vi "results.vi"(11 "Quantities":T1[](array[typedef])) -> (3 "Quantities out":T1[](array[typedef]))   [LabVIEW 2013]
uses:
  qwtb_lvlib/TD Quantity.ctl
  <vilib>/Utility/xml.llb/Write to XML File(string).vi
  <vilib>/Utility/xml.llb/Read From XML File(string).vi
panel:
  in  "load Q":bool
  in  "save Q":bool
  in  "Q list curr value":i32
  in  "Q list":i32(listbox) caption="Input Quantities"
  in  "quit":bool
  out "Q name":string caption="Name of Quantity:"
  in  "Q type":enum32{"Scalar", "Vector"}(tab)
  out "scalar dof":dbl=1.0 caption="DoF"
  out "scalar value":dbl=1.0 caption="Value"
  out "scalar unc":dbl=1.0 caption="Uncertainty"
  in  "set dof same as 1st":bool
  out "vector dof":dbl[](array[numeric]) caption="DoF"
  out "vector value":dbl[](array[numeric]) caption="Value"
  out "vector unc":dbl[](array[numeric]) caption="Uncertainty"
  out "Value Graph":dbl[](graph)
  in  "load csv":bool
  # "Results"
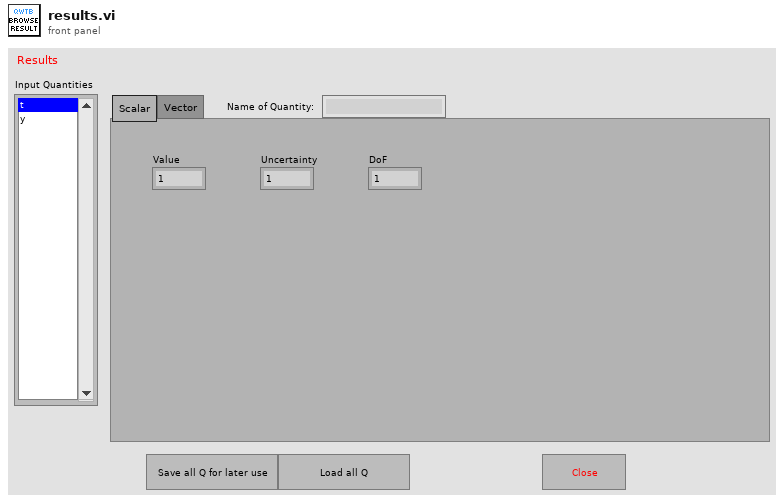
[diagram p1: front panel]
types:
  T1 = typedef "TD Quantity.ctl" = cluster{"Name":string, "Value":dbl[], "Uncertainty":dbl[][], "Degrees of\nFreedom":dbl[]}
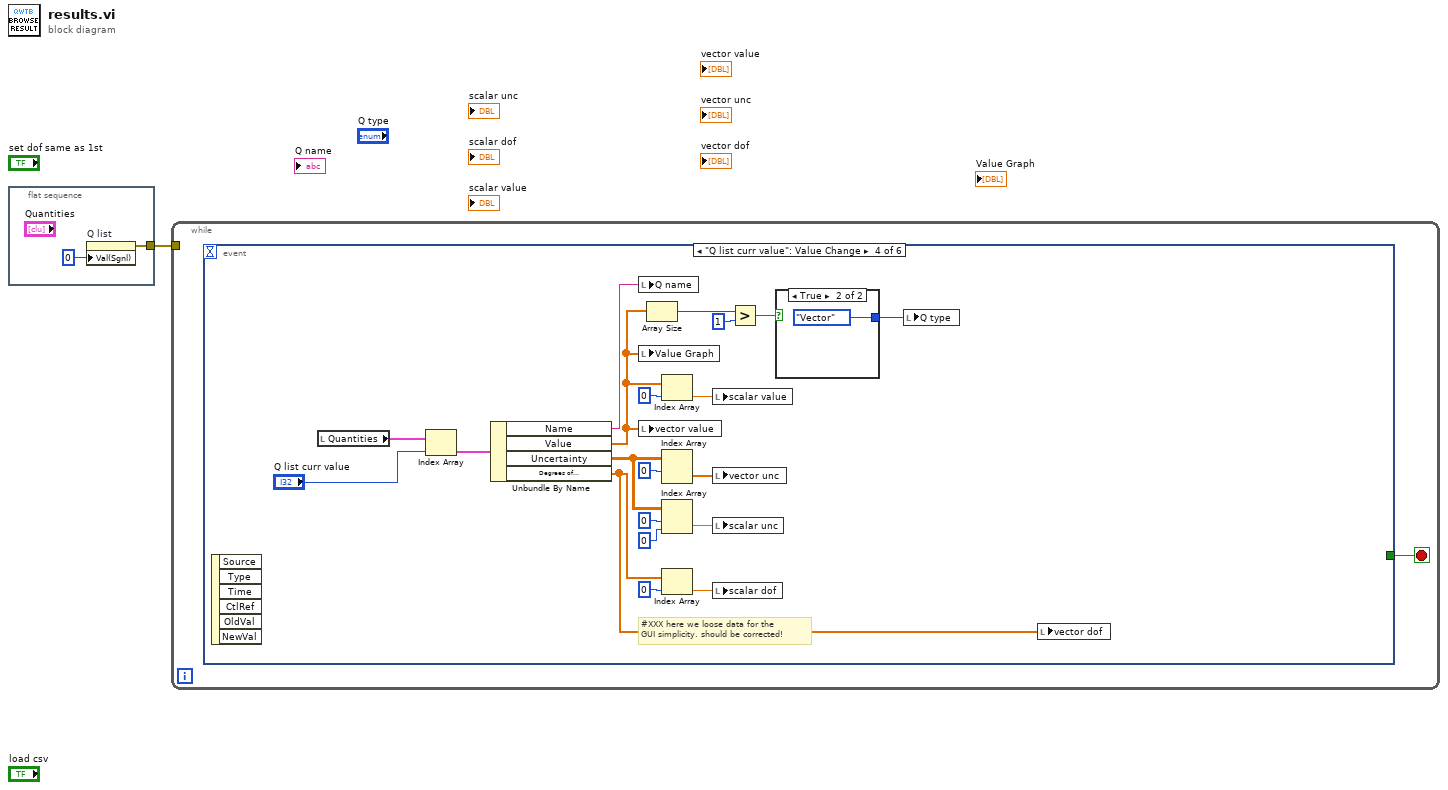
[diagram p0: block diagram]
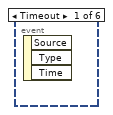
[diagram p2: hidden frame]
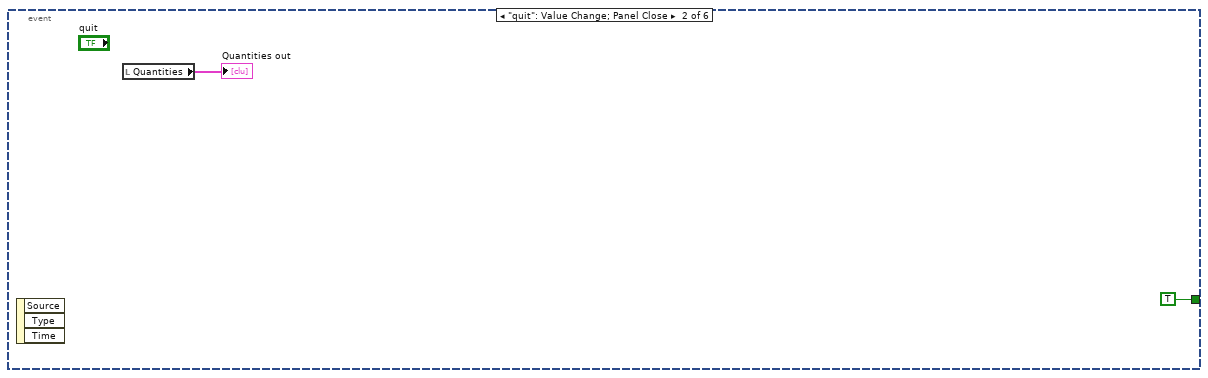
[diagram p3: hidden frame]
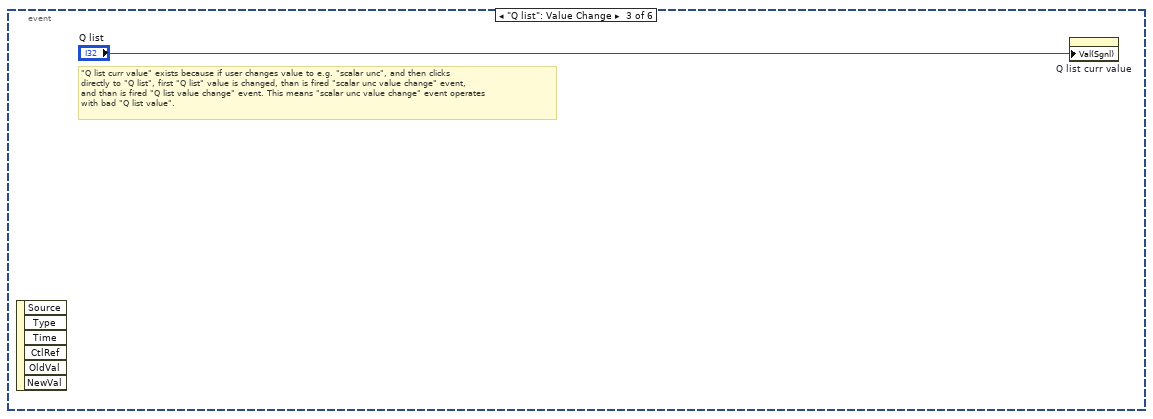
[diagram p4: hidden frame]
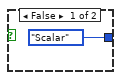
[diagram p5: hidden frame]
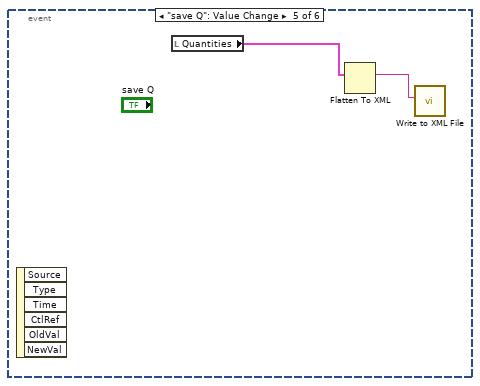
[diagram p6: hidden frame]
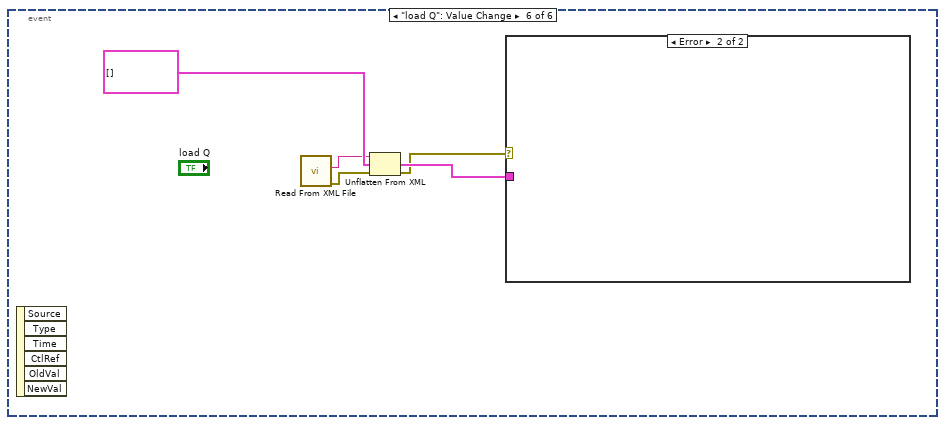
[diagram p7: hidden frame]
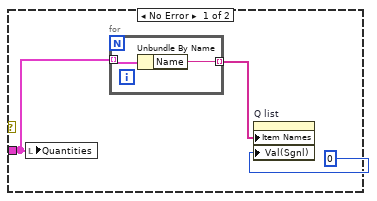
[diagram p8: hidden frame]
diagram:
  n1 = flat-sequence {
    tunnel: [w2] -> w1
    frame #0 {
      n2 = property on="Q list" class="LstBox (strict)"("Val(Sgnl)"=0 ("Value (Signaling)")) -> (error out=w2:errorcluster)  [unwired: 2 in, 1 out]
    }
  }
  n3 = while {
    tunnel: w1 -> [_]
    stop <- w4 stop-if-true
    n4 = event shown="[3] \"Q list curr value\": Value Change" {
      selector: _ -> [_ _ _ _ _ _]
      dyn-events: _ -> [_ _ _ _ _ _]
      timeout: _ -> [_ _ _ _ _ _]
      tunnel: [_ TRUE _ _ _ _] -> w4
      event Timeout {
        n5 = event-data() -> ()  [unwired: 1 in, 3 out]
      }
      event "quit": Value Change; Panel Close {
        n6 = event-data() -> ()  [unwired: 1 in, 3 out]
        n7 = local read "Quantities"() -> (→"Quantities out":T1[])
      }
      event "Q list": Value Change {
        # "\"Q list curr value\" exists because if user changes value to e.g. \"scalar unc\", and then clicks\ndirectly to \"Q list\", first \"Q list\" value is changed, than is fired \"scalar unc value change\" event,\nand than is fired \"Q list value change\" event. This means \"scalar unc value change\" event operates\nwith bad \"Q list value\"."
        n8 = event-data() -> ()  [unwired: 1 in, 6 out]
        n9 = property on="Q list curr value" class="DigNum (strict)"("Val(Sgnl)"="Q list") -> ()  [unwired: 2 in, 2 out]
      }
      event "Q list curr value": Value Change {
        # "#XXX here we loose data for the\nGUI simplicity. should be corrected!"
        n10 = event-data() -> ()  [unwired: 1 in, 6 out]
        n11 = local read "Quantities"() -> (w25:T1[])
        n12 = Index Array(array=w25, index="Q list curr value") -> (element=w27:T1)
        n13 = Unbundle By Name(w27) -> ("Name"=w26:string, "Value"=w11:dbl[], "Uncertainty"=w12:dbl[][], "Degrees of\nFreedom"=w8:dbl[])
        n14 = local write "Q name"(w26) -> ()
        n15 = local write "Value Graph"(w11) -> ()
        n16 = local write "vector value"(w11) -> ()
        n17 = Array Size(array=w11) -> (size(s)=w24:i32)
        n18 = Index Array(array=w11, index=0) -> (element=w13:dbl)
        n19 = Index Array(array=w12, index (row)=0) -> (element=w19:dbl[])  [unwired: 1 in]
        n20 = Index Array(array=w12, index (row)=0, index (col)=0 ("disabled index (col)")) -> (element=w16:dbl)
        n21 = Index Array(array=w8, index=0) -> (element=w9:dbl)
        n22 = local write "scalar value"(w13) -> ()
        n23 = local write "vector unc"(w19) -> ()
        n24 = local write "scalar unc"(w16) -> ()
        n25 = local write "scalar dof"(w9) -> ()
        n26 = Greater?(x=w24, y=1) -> (0:w22:bool)
        n27 = case shown="True" w22 {
          tunnel: [enum32{"Scalar", "Vector"}."Scalar" ("Quantity type") enum32{"Scalar", "Vector"}."Vector" ("Quantity type")] -> w21
          frame False {
          }
          frame True {
          }
        }
        n28 = local write "Q type"(w21) -> ()
        n29 = local write "vector dof"(w8) -> ()
      }
      event "save Q": Value Change {
        n30 = event-data() -> ()  [unwired: 1 in, 6 out]
        n31 = local read "Quantities"() -> (w31:T1[])
        n32 = Flatten To XML(anything=w31) -> (xml string=w30:string)
        n33 = call-poly <vilib>:"Write to XML File.vi"("XML Input"=w30) -> ()  [unwired: 8 in, 3 out]
      }
      event "load Q": Value Change {
        n34 = event-data() -> ()  [unwired: 1 in, 6 out]
        n35 = call-poly <vilib>:"Read From XML File.vi"() -> ("error out"=w36:errorcluster, "XML Elements"=w34:string)  [unwired: 9 in, 1 out]
        n36 = Unflatten From XML(xml string=w34, type=T1[] [], error in (no error)=w36) -> (value=w33:T1[], error out=w32:errorcluster)
        n37 = case shown="Error" w32 {
          tunnel: w33 -> [w39 _]
          frame No Error {
            n38 = local write "Quantities"(w39) -> ()
            n39 = for {
              tunnel: w39 -> [w41] mode=indexing
              tunnel: [w40] -> w37 mode=indexing
              n40 = Unbundle By Name(w41) -> ("Name"=w40:string)
            }
            n41 = property on="Q list" class="LstBox (strict)"("Item Names"=w37, "Val(Sgnl)"=0 ("Value (Signaling)")) -> ()  [unwired: 2 in, 2 out]
          }
          frame Error {
          }
        }
      }
    }
  }
